vi "load_xml.vi"(8 "error in":errorcluster, 10 "child node in":refnum<k20>, 11 "Analog_Output.lvclass (in)":refnum<class "Analog_Output.lvclass">) -> (0 "error out":errorcluster, 2 "child node out":refnum<k20>, 3 "Analog_Output.lvclass":refnum<class "Analog_Output.lvclass">)   [LabVIEW 2013, in "Analog_Output.lvclass"]
doc: "Loads analog output settings from xml. Expected format:\n\n<Enable>%b</Enable>\n<PhysicalChannel>%s</PhysicalChannel>\n<MinimumValue>%f</MinimumValue>\n<MaximumValue>%f</MaximumValue>\n<SamplesPerSecond>%f</SamplesPerSecond>\n<TotalAOTime units=\"seconds\">%s</TotalAOTime>\n<AnalogOutputEquations>\n%s</AnalogOutputEquations>\n<StartTrigger.WaitForStartTrigger>%b</StartTrigger.WaitForStartTrigger\n<StartTrigger.source>%s</StartTrigger.source>\n<StartTrigger.edge>%s</StartTrigger.edge>\n\nMTL 2012 Dec 31"
uses:
  Analog_Output.lvclass
  Analog_Output.lvclass/Analog_Output.ctl
  Experiment/Globals.vi
  <vilib>/xml/Close Reference(Node).vi
  <resource>/objmgr/DOMUserDefRef.rc
  <vilib>/xml/NI_XML.lvlib
panel:
  out "size(s)":i32[](array[numeric])
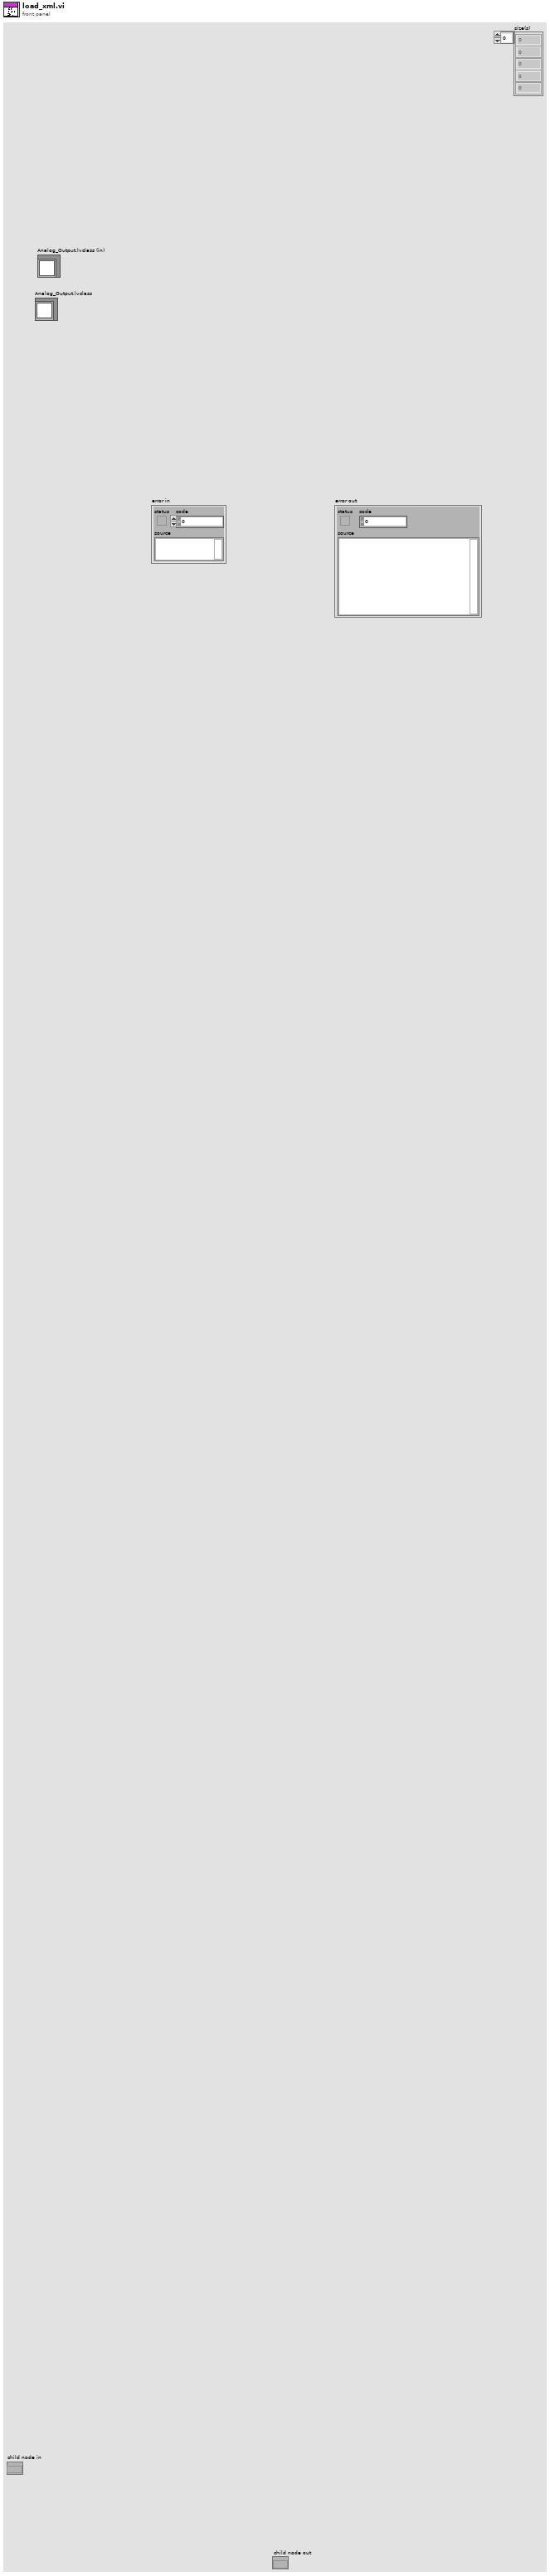
[diagram p1: front panel]
types:
  T1 = typedef "Analog_Output.lvclass/AO_settings.ctl" = cluster{"Enable Analog Out?":bool, "Physical Channel":tag, "Minimum Value":dbl, "Maximum Value":dbl, "Samples per second":dbl, "Total AO Time (seconds)":dbl, "Start Trigger":cluster{"Wait for start trigger?":bool, "source":tag, "edge":i32}, "Analog Output Waveforms (channel, time)":dbl[][], "Export trigger":cluster{"Export Start Trigger?":bool, "output terminal":tag}}
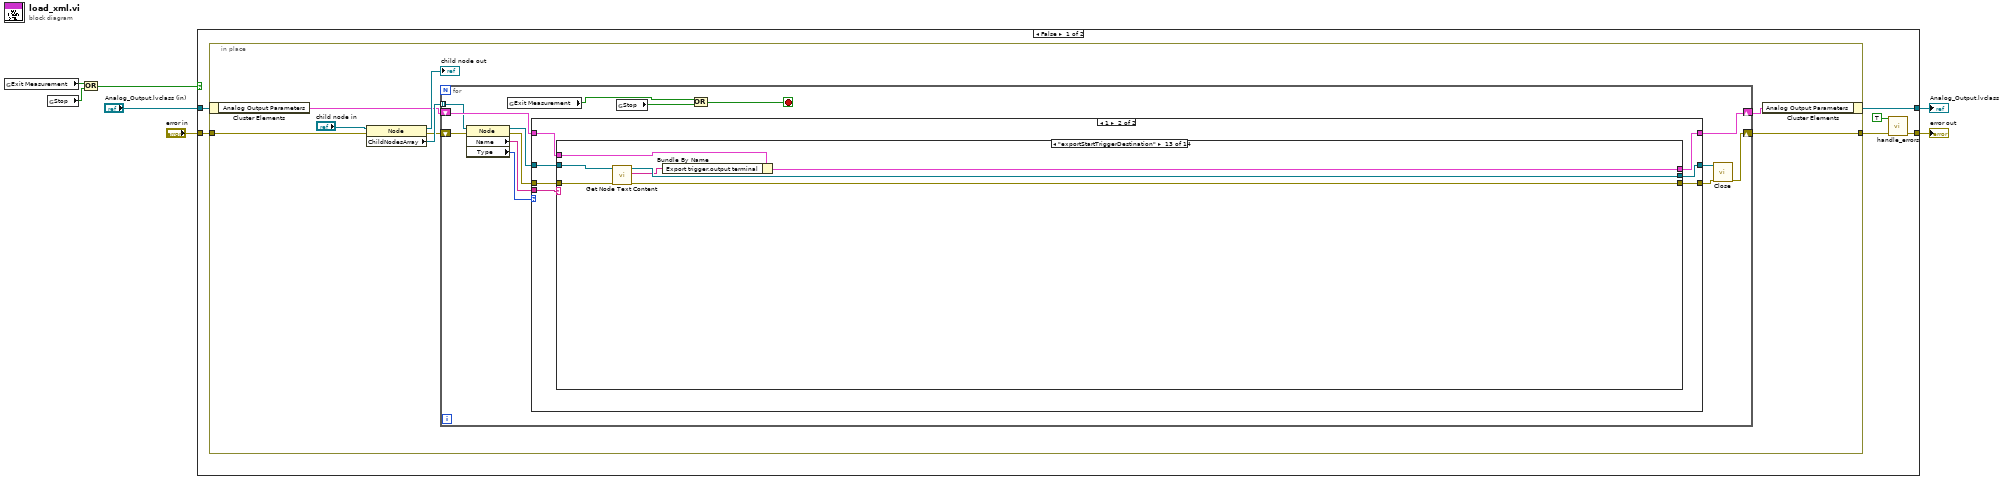
[diagram p0: block diagram]
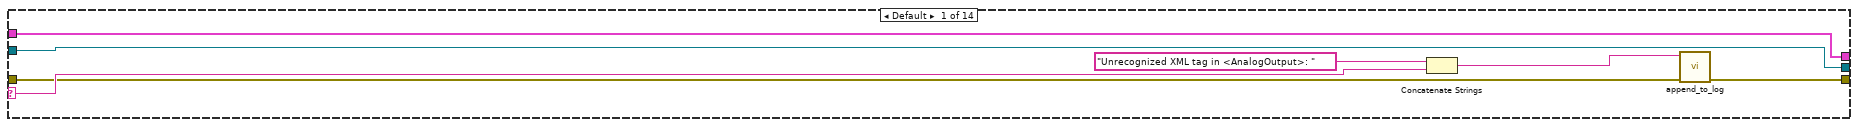
[diagram p3: hidden frame]
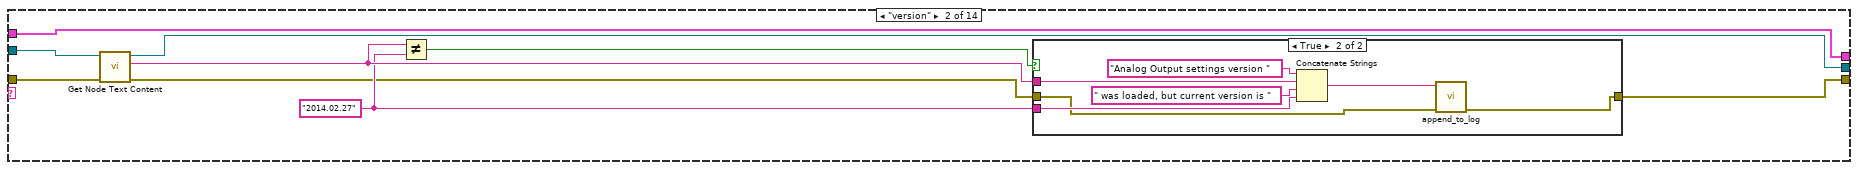
[diagram p4: hidden frame]
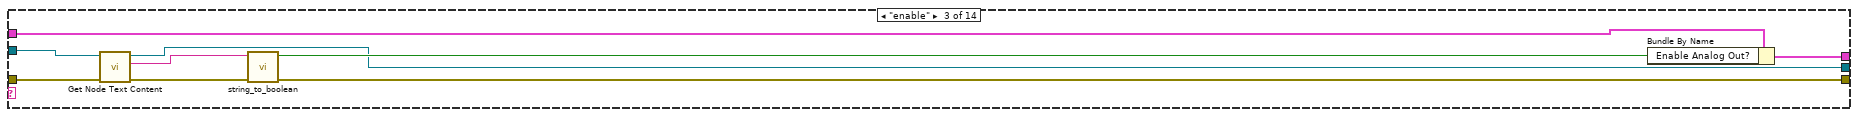
[diagram p6: hidden frame]
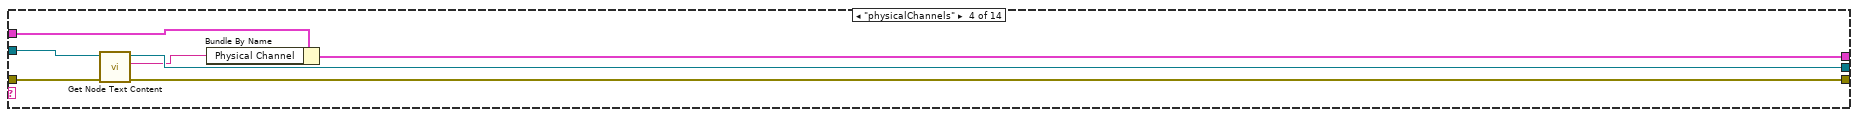
[diagram p7: hidden frame]
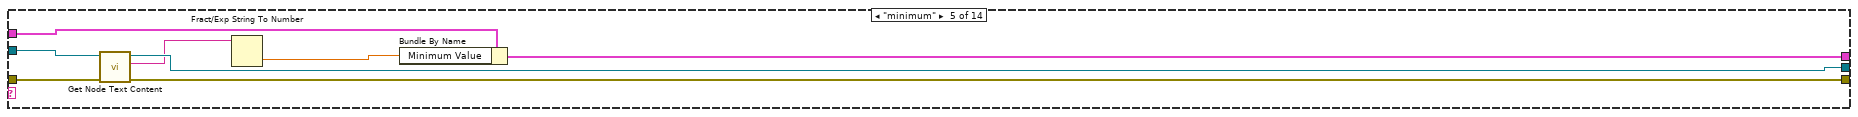
[diagram p8: hidden frame]
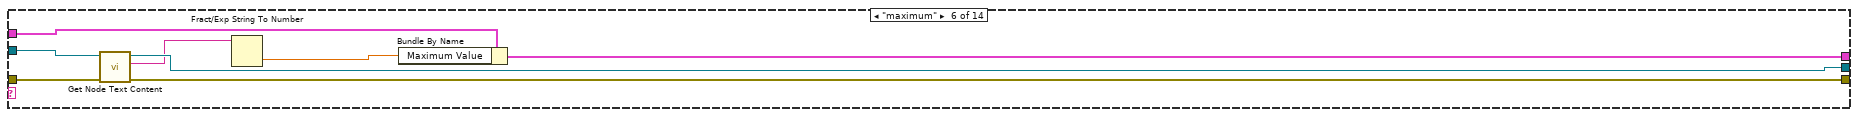
[diagram p9: hidden frame]
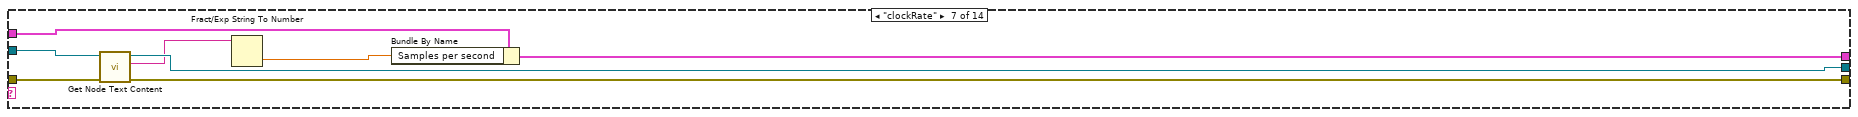
[diagram p10: hidden frame]
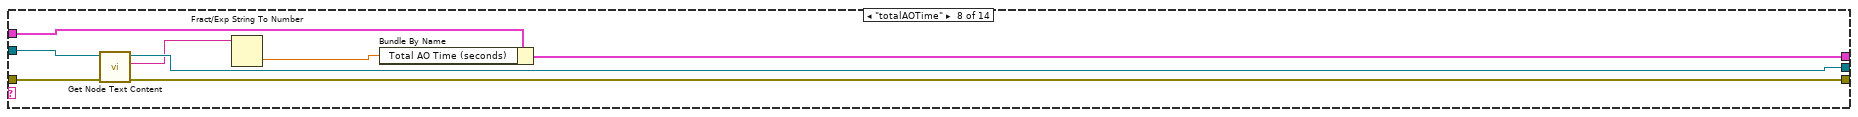
[diagram p11: hidden frame]
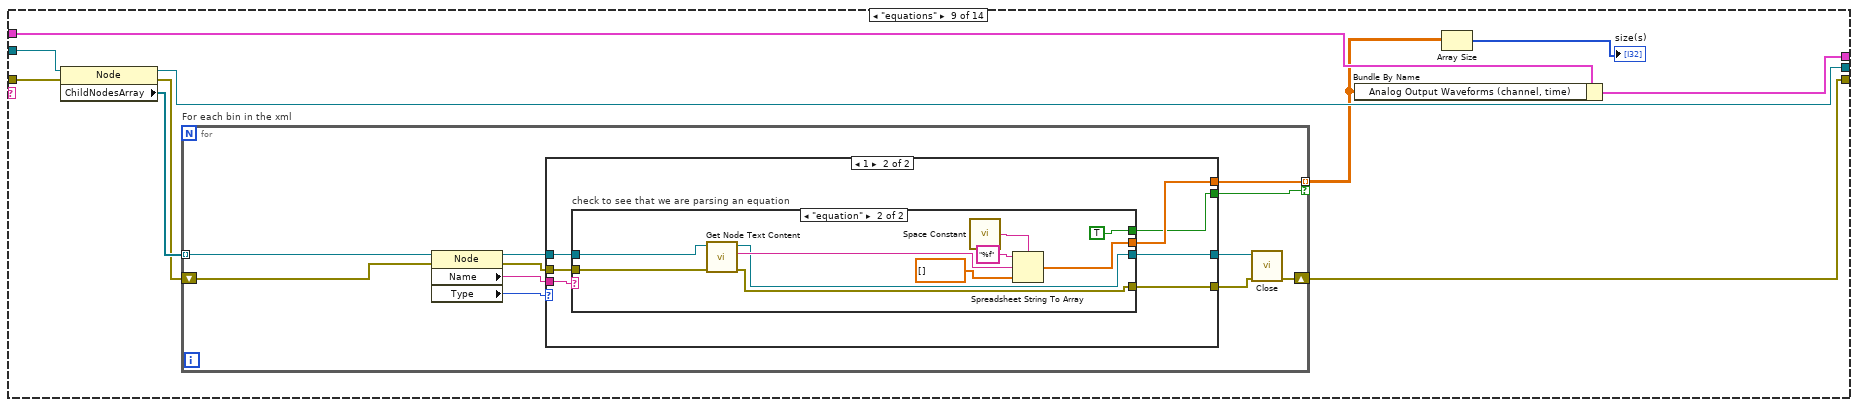
[diagram p12: hidden frame]
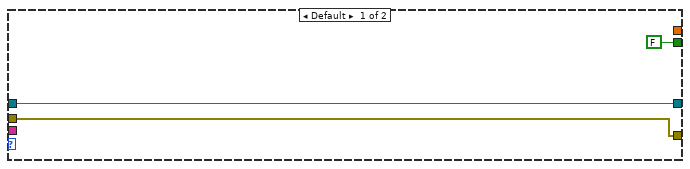
[diagram p13: hidden frame]
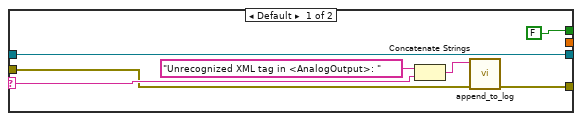
[diagram p14: hidden frame]
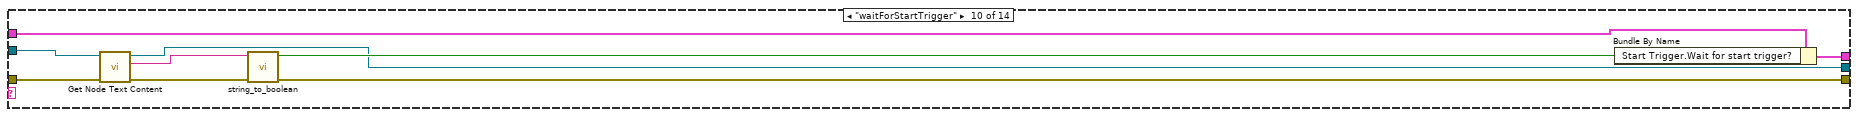
[diagram p15: hidden frame]
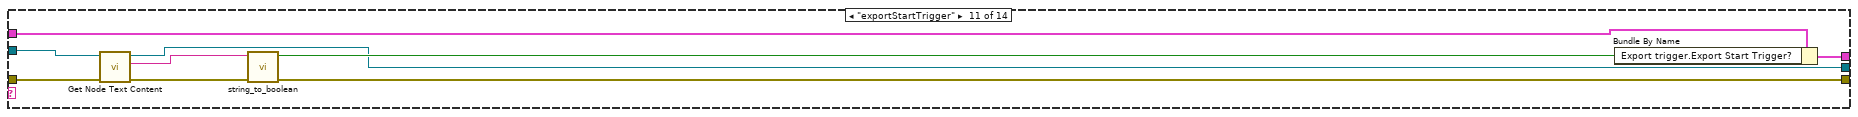
[diagram p16: hidden frame]
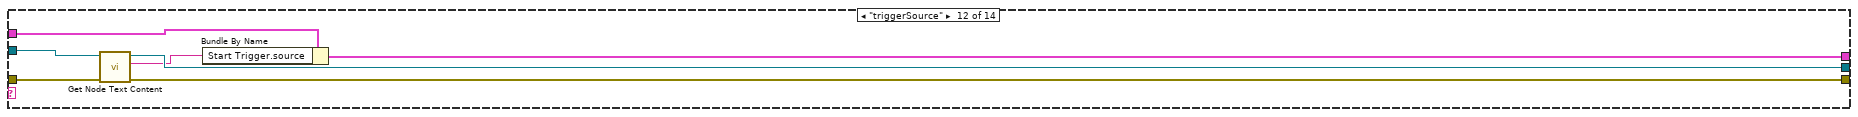
[diagram p17: hidden frame]
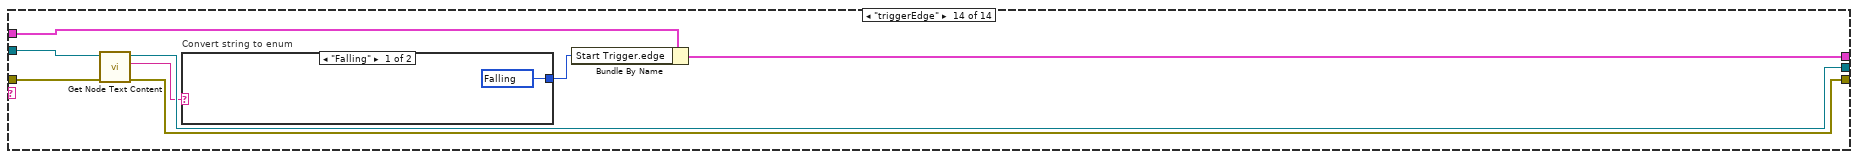
[diagram p18: hidden frame]
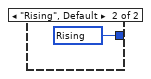
[diagram p19: hidden frame]
diagram:
  n1 = global read "Globals.vi" "Exit Measurement"() -> (w4:bool)
  n2 = global read "Globals.vi" "Stop"() -> (w3:bool)
  n3 = Or(x=w4, y=w3) -> (x .or. y?=w2:bool)
  n4 = case shown="False" w2 {
    tunnel: "Analog_Output.lvclass (in)" -> [w13 w208]
    tunnel: [w12 w208] -> w6
    tunnel: "error in" -> [w11 w209]
    tunnel: [w8 w209] -> w1
    frame False {
      n5 = in-place {
        in-place-border: w11 -> [w15]
        in-place-border: [w14] -> w10
        n6 = in-place-cluster #1(w13) -> ("Analog Output Parameters"=w16:T1)
        n7 = property class="Node"(reference="child node in", error in=w15) -> (reference out=→"child node out":refnum<k20>, error out=w19:errorcluster, "ChildNodesArray"=w21:refnum<k20>[])
        n8 = for {
          tunnel: w21 -> [w26] mode=indexing
          shift-right: [w32] -> w17
          shift-left: w16 -> [w33]
          shift-right: [w29] -> w14
          shift-left: w19 -> [w27]
          stop <- w22 stop-if-true
          n9 = property class="Node"(reference=w26, error in=w27) -> (reference out=w34:refnum<k20>, error out=w30:errorcluster, "Name"=w35:string, "Type"=w25:i32)
          n10 = global read "Globals.vi" "Exit Measurement"() -> (w24:bool)
          n11 = case shown="1" w25 {
            tunnel: w35 -> [_ w45]
            tunnel: w34 -> [w38 w44]
            tunnel: w33 -> [w36 w43]
            tunnel: [w36 w42] -> w32
            tunnel: [w38 w41] -> w31
            tunnel: w30 -> [w37 w40]
            tunnel: [w37 w39] -> w28
            frame Default {
            }
            frame 1 {
              n12 = case shown="\"exportStartTriggerDestination\"" w45 {
                selector: w45 -> [w48 _ _ _ _ _ _ _ _ _ _ _ _ _]
                tunnel: w44 -> [w51 w55 w78 w85 w93 w101 w109 w117 w125 w174 w183 w190 w197 w205]
                tunnel: w43 -> [w52 w57 w76 w83 w91 w99 w107 w115 w127 w172 w181 w188 w195 w203]
                tunnel: [w52 w57 w75 w82 w90 w98 w106 w114 w126 w171 w180 w187 w194 w202] -> w42
                tunnel: [w51 w54 w70 w81 w89 w97 w105 w113 w122 w166 w175 w186 w193 w201] -> w41
                tunnel: w40 -> [w47 w56 w77 w84 w92 w100 w108 w116 w121 w173 w182 w189 w196 w204]
                tunnel: [w46 w53 w73 w79 w88 w96 w104 w112 w120 w169 w178 w184 w191 w200] -> w39
                frame Default {
                  n13 = Concatenate Strings("Unrecognized XML tag in <AnalogOutput>: " ("string"), w48) -> (w49:string)
                  n14 = call "append_to_log.vi"("error in"=w47, "string"=w49) -> ("error out"=w46:errorcluster)  [unwired: 9 in]
                }
                frame "version" {
                  w59 = "2014.02.27" ("y")
                  n15 = call <vilib>:"Get Node Text Content.vi"("error in (no error)"=w56, "node in"=w55) -> ("error out"=w58:errorcluster, "node text"=w60:string, "node out"=w54:refnum<k20>)  [unwired: 7 in]
                  n16 = Not Equal?(x=w60, y=w59) -> (x != y?=w61:bool)
                  n17 = case shown="True" w61 {
                    tunnel: w60 -> [_ w68]
                    tunnel: w59 -> [_ w66]
                    tunnel: w58 -> [w62 w64]
                    tunnel: [w62 w63] -> w53
                    frame False {
                    }
                    frame True {
                      n18 = Concatenate Strings("Analog Output settings version " ("string"), w68, " was loaded, but current version is " ("string"), w66) -> (w65:string)
                      n19 = call "append_to_log.vi"("error in"=w64, "string"=w65) -> ("error out"=w63:errorcluster)  [unwired: 9 in]
                    }
                  }
                }
                frame "enable" {
                  n20 = call <vilib>:"Get Node Text Content.vi"("error in (no error)"=w77, "node in"=w78) -> ("error out"=w74:errorcluster, "node text"=w72:string, "node out"=w70:refnum<k20>)  [unwired: 7 in]
                  n21 = call "string_to_boolean.vi"("error in"=w74, "string"=w72) -> ("error out"=w73:errorcluster, "boolean"=w71:bool)  [unwired: 8 in]
                  n22 = Bundle By Name(cluster=w76, "Enable Analog Out?"=w71) -> (w75:T1)
                }
                frame "physicalChannels" {
                  n23 = call <vilib>:"Get Node Text Content.vi"("error in (no error)"=w84, "node in"=w85) -> ("error out"=w79:errorcluster, "node text"=w80:string, "node out"=w81:refnum<k20>)  [unwired: 7 in]
                  n24 = Bundle By Name(cluster=w83, "Physical Channel"=w80) -> (w82:T1)
                }
                frame "minimum" {
                  n25 = call <vilib>:"Get Node Text Content.vi"("error in (no error)"=w92, "node in"=w93) -> ("error out"=w88:errorcluster, "node text"=w87:string, "node out"=w89:refnum<k20>)  [unwired: 7 in]
                  n26 = Fract/Exp String To Number(string=w87) -> (number=w86:dbl)  [unwired: 3 in, 1 out]
                  n27 = Bundle By Name(cluster=w91, "Minimum Value"=w86) -> (w90:T1)
                }
                frame "maximum" {
                  n28 = call <vilib>:"Get Node Text Content.vi"("error in (no error)"=w100, "node in"=w101) -> ("error out"=w96:errorcluster, "node text"=w95:string, "node out"=w97:refnum<k20>)  [unwired: 7 in]
                  n29 = Fract/Exp String To Number(string=w95) -> (number=w94:dbl)  [unwired: 3 in, 1 out]
                  n30 = Bundle By Name(cluster=w99, "Maximum Value"=w94) -> (w98:T1)
                }
                frame "clockRate" {
                  n31 = call <vilib>:"Get Node Text Content.vi"("error in (no error)"=w108, "node in"=w109) -> ("error out"=w104:errorcluster, "node text"=w103:string, "node out"=w105:refnum<k20>)  [unwired: 7 in]
                  n32 = Fract/Exp String To Number(string=w103) -> (number=w102:dbl)  [unwired: 3 in, 1 out]
                  n33 = Bundle By Name(cluster=w107, "Samples per second"=w102) -> (w106:T1)
                }
                frame "totalAOTime" {
                  n34 = call <vilib>:"Get Node Text Content.vi"("error in (no error)"=w116, "node in"=w117) -> ("error out"=w112:errorcluster, "node text"=w111:string, "node out"=w113:refnum<k20>)  [unwired: 7 in]
                  n35 = Fract/Exp String To Number(string=w111) -> (number=w110:dbl)  [unwired: 3 in, 1 out]
                  n36 = Bundle By Name(cluster=w115, "Total AO Time (seconds)"=w110) -> (w114:T1)
                }
                frame "equations" {
                  n37 = property class="Node"(reference=w125, error in=w121) -> (reference out=w122:refnum<k20>, error out=w123:errorcluster, "ChildNodesArray"=w124:refnum<k20>[])
                  n38 = for "For each bin in the xml" {
                    shift-right: [w128] -> w120
                    shift-left: w123 -> [w136]
                    tunnel: w124 -> [w138] mode=indexing
                    tunnel: [w134] -> w119 mode=indexing if=w133
                    n39 = property class="Node"(reference=w138, error in=w136) -> (reference out=w137:refnum<k20>, error out=w135:errorcluster, "Name"=w132:string, "Type"=w131:i32)
                    n40 = case shown="1" w131 {
                      tunnel: w137 -> [w139 w148]
                      tunnel: w135 -> [w140 w147]
                      tunnel: [_ w146] -> w134
                      tunnel: [FALSE w145] -> w133
                      tunnel: [w140 w144] -> w129
                      tunnel: w132 -> [_ w143]
                      tunnel: [w139 w142] -> w130
                      frame Default {
                      }
                      frame 1 {
                        n41 = case "check to see that we are parsing an equation" shown="\"equation\"" w143 {
                          selector: w143 -> [w152 _]
                          tunnel: w148 -> [w149 w165]
                          tunnel: w147 -> [w151 w164]
                          tunnel: [_ w160] -> w146
                          tunnel: [FALSE TRUE] -> w145
                          tunnel: [w150 w158] -> w144
                          tunnel: [w149 w156] -> w142
                          frame Default {
                            n42 = Concatenate Strings("Unrecognized XML tag in <AnalogOutput>: " ("string"), w152) -> (w153:string)
                            n43 = call "append_to_log.vi"("error in"=w151, "string"=w153) -> ("error out"=w150:errorcluster)  [unwired: 9 in]
                          }
                          frame "equation" {
                            n44 = call <vilib>:"Get Node Text Content.vi"("error in (no error)"=w164, "node in"=w165) -> ("error out"=w158:errorcluster, "node text"=w157:string, "node out"=w156:refnum<k20>)  [unwired: 7 in]
                            n45 = call <vilib>:"Space Constant.vi"() -> ("String"=w161:string)
                            n46 = Spreadsheet String To Array(delimiter (Tab)=w161, format string="%f", spreadsheet string=w157, array type (2D Dbl)=dbl[] []) -> (array=w160:dbl[])
                          }
                        }
                      }
                    }
                    n47 = call-poly <vilib>:"Close.vi"("error in (no error)"=w129, "node"=w130) -> ("error out"=w128:errorcluster)  [unwired: 7 in]
                  }
                  n48 = Bundle By Name(cluster=w127, "Analog Output Waveforms (channel, time)"=w119) -> (w126:T1)
                  n49 = Array Size(array=w119) -> (size(s)=→"size(s)":i32[])
                }
                frame "waitForStartTrigger" {
                  n50 = call <vilib>:"Get Node Text Content.vi"("error in (no error)"=w173, "node in"=w174) -> ("error out"=w170:errorcluster, "node text"=w168:string, "node out"=w166:refnum<k20>)  [unwired: 7 in]
                  n51 = call "string_to_boolean.vi"("error in"=w170, "string"=w168) -> ("error out"=w169:errorcluster, "boolean"=w167:bool)  [unwired: 8 in]
                  n52 = Bundle By Name(cluster=w172, "Start Trigger.Wait for start trigger?"=w167) -> (w171:T1)
                }
                frame "exportStartTrigger" {
                  n53 = call <vilib>:"Get Node Text Content.vi"("error in (no error)"=w182, "node in"=w183) -> ("error out"=w179:errorcluster, "node text"=w177:string, "node out"=w175:refnum<k20>)  [unwired: 7 in]
                  n54 = call "string_to_boolean.vi"("error in"=w179, "string"=w177) -> ("error out"=w178:errorcluster, "boolean"=w176:bool)  [unwired: 8 in]
                  n55 = Bundle By Name(cluster=w181, "Export trigger.Export Start Trigger?"=w176) -> (w180:T1)
                }
                frame "triggerSource" {
                  n56 = call <vilib>:"Get Node Text Content.vi"("error in (no error)"=w189, "node in"=w190) -> ("error out"=w184:errorcluster, "node text"=w185:string, "node out"=w186:refnum<k20>)  [unwired: 7 in]
                  n57 = Bundle By Name(cluster=w188, "Start Trigger.source"=w185) -> (w187:T1)
                }
                frame "exportStartTriggerDestination" {
                  n58 = call <vilib>:"Get Node Text Content.vi"("error in (no error)"=w196, "node in"=w197) -> ("error out"=w191:errorcluster, "node text"=w192:string, "node out"=w193:refnum<k20>)  [unwired: 7 in]
                  n59 = Bundle By Name(cluster=w195, "Export trigger.output terminal"=w192) -> (w194:T1)
                }
                frame "triggerEdge" {
                  n60 = call <vilib>:"Get Node Text Content.vi"("error in (no error)"=w204, "node in"=w205) -> ("error out"=w200:errorcluster, "node text"=w199:string, "node out"=w201:refnum<k20>)  [unwired: 7 in]
                  n61 = case "Convert string to enum" shown="\"Falling\"" w199 {
                    tunnel: [w206 w207] -> w198
                    frame "Falling" {
                      w206 = 10171 items=["Rising"=10280, "Falling"=10171] ("edge")
                    }
                    frame "Rising", Default {
                      w207 = 10280 items=["Rising"=10280, "Falling"=10171] ("edge")
                    }
                  }
                  n62 = Bundle By Name(cluster=w203, "Start Trigger.edge"=w198) -> (w202:T1)
                }
              }
            }
          }
          n63 = global read "Globals.vi" "Stop"() -> (w23:bool)
          n64 = Or(x=w24, y=w23) -> (x .or. y?=w22:bool)
          n65 = call-poly <vilib>:"Close.vi"("error in (no error)"=w28, "node"=w31) -> ("error out"=w29:errorcluster)  [unwired: 7 in]
        }
        n66 = in-place-cluster #1("Analog Output Parameters"=w17) -> (w12:refnum<class "Analog_Output.lvclass">)
      }
      n67 = call "handle_errors.vi"("Exit Operation"=TRUE, "error in (no error)"=w10) -> ("error out"=w8:errorcluster)  [unwired: 13 in]
    }
    frame True {
    }
  }
  "Analog_Output.lvclass" <- w6
  "error out" <- w1
